vi "loadDataPerChannel.vi"(8 "error in (no error)":errorcluster, 10 "data":dbl[][][](array[numeric]), 11 "K2602 in":refnum<class "K2602.lvclass">) -> (0 "error out":errorcluster, 3 "K2602 out":refnum<class "K2602.lvclass">)   [LabVIEW 2009, in "Hardware.lvlib" / "Channels.lvlib" / "K2602.lvclass"]
uses:
  K2602.lvclass
  K2602.lvclass/K2602.ctl
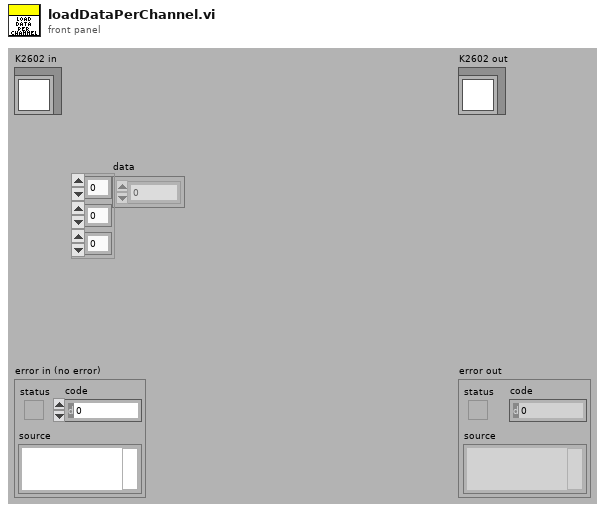
[diagram p1: front panel]
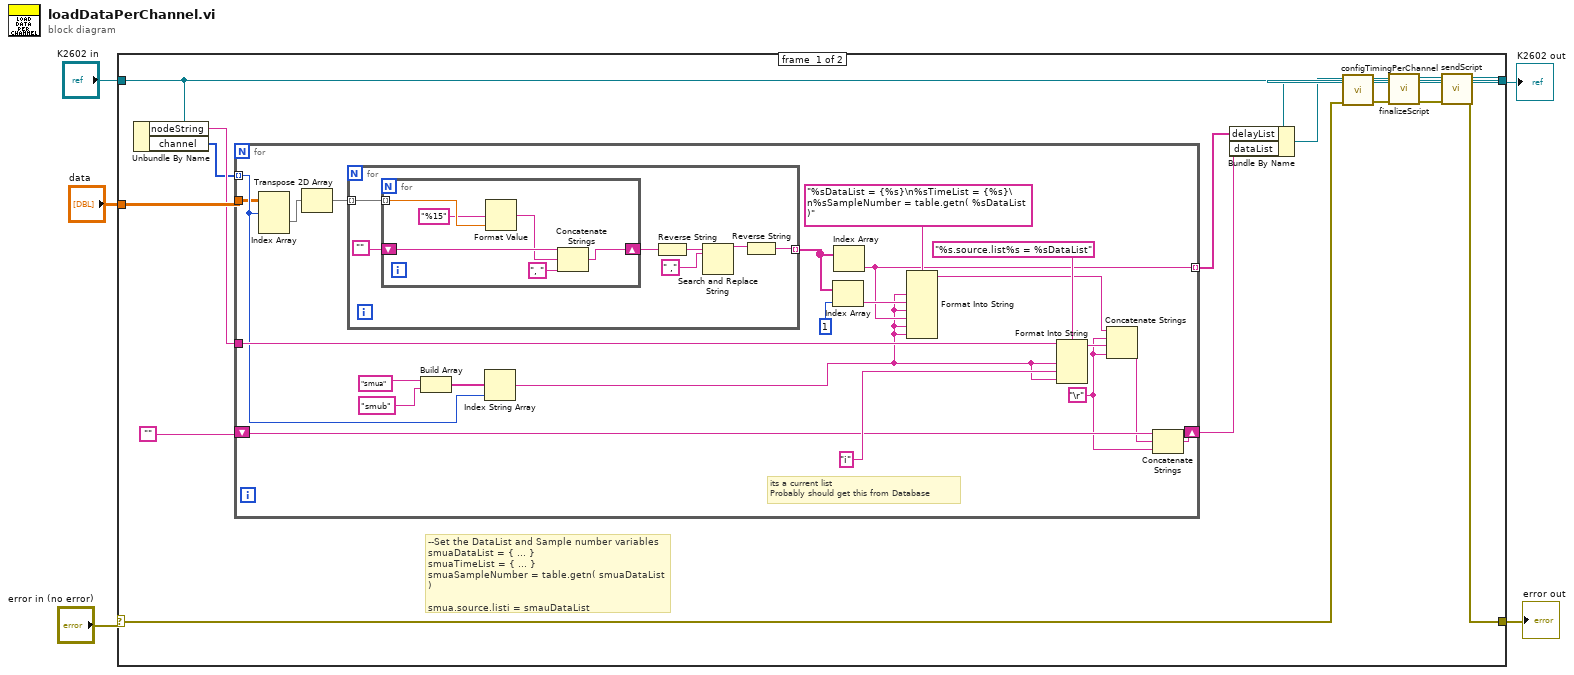
[diagram p0: block diagram]
diagram:
  n1 = case shown="No Error" "error in (no error)" {
    selector: "error in (no error)" -> [w13 w56]
    tunnel: [w7 w56] -> w4
    tunnel: [w8 w57] -> w2
    tunnel: "K2602 in" -> [w18 w57]
    tunnel: "data" -> [w20 _]
    frame #0 {
      # "--Set the DataList and Sample number variables\nsmuaDataList = { ... }\nsmuaTimeList = { ... }\nsmuaSampleNumber = table.getn( smuaDataList ) \n\nsmua.source.listi = smauDataList"
      n2 = Unbundle By Name(w18) -> ("nodeString"=w19:string, "channel"=w6:i32[])
      n3 = for {
        tunnel: w20 -> [w22]
        tunnel: w19 -> [w39]
        tunnel: [w27] -> w17 mode=indexing
        shift-right: [w34] -> w15
        shift-left: "" -> [w33]
        tunnel: w6 -> [w23] mode=indexing
        w24 = "\r"
        # "its a current list\nProbably should get this from Database"
        n4 = Index Array(array=w22, index (dim 0)=w23) -> (element=w21:dbl[][])  [unwired: 2 in]
        n5 = Transpose 2D Array(2D array=w21) -> (transposed array=w25:dbl[][])
        n6 = for {
          tunnel: w25 -> [w49] mode=indexing
          tunnel: [w43] -> w35 mode=indexing
          n7 = for {
            tunnel: w49 -> [w55] mode=indexing
            shift-right: [w50] -> w47
            shift-left: "" -> [w53]
            n8 = Format Value(format string="%15", value (0)=w55) -> (output string=w52:string)  [unwired: 1 in]
            n9 = Concatenate Strings(w53, w52, ", ") -> (w50:string)
          }
          n10 = Reverse String(1:w47) -> (0:w46:string)
          n11 = Search and Replace String(input string=w46, search string=" ,") -> (result string=w44:string)  [unwired: 6 in, 3 out]
          n12 = Reverse String(1:w44) -> (0:w43:string)
        }
        n13 = Build Array("smua", "smub") -> (w40:string[])
        n14 = Index String Array(1:w23, 2:w40) -> (0:w26:string)  [unwired: 1 in]
        n15 = Index Array(array=w35, index=1) -> (element=w31:string)
        n16 = Index Array(array=w35) -> (element=w27:string)  [unwired: 1 in]
        n17 = Format Into String(format string="%sDataList = {%s}\n%sTimeList = {%s}\n%sSampleNumber = table.getn( %sDataList )", w26, w31, w26, w27, w26, w26) -> (resulting string=w29:string)  [unwired: 2 in, 1 out]
        n18 = Format Into String(format string="%s.source.list%s = %sDataList", initial string=w39, w26, "i", w26) -> (resulting string=w28:string)  [unwired: 1 in, 1 out]
        n19 = Concatenate Strings(w29, w24, w28, w24) -> (w32:string)
        n20 = Concatenate Strings(w33, w32, w24) -> (w34:string)
      }
      n21 = Bundle By Name(cluster=w18, "delayList"=w17, "dataList"=w15) -> (w14:refnum<class "K2602.lvclass">)
      n22 = call-dynamic "configTimingPerChannel.vi"("error in (no error)"=w13, "K2602 in"=w14) -> ("error out"=w11:errorcluster, "K2602 out"=w12:refnum<class "K2602.lvclass">)  [unwired: 8 in]
      n23 = call "finalizeScript.vi"("error in (no error)"=w11, "K2602 in"=w12) -> ("error out"=w9:errorcluster, "K2602 out"=w10:refnum<class "K2602.lvclass">)  [unwired: 7 in, 1 out]
      n24 = call "sendScript.vi"("error in (no error)"=w9, "K2602 in"=w10) -> ("error out"=w7:errorcluster, "K2602 out"=w8:refnum<class "K2602.lvclass">)  [unwired: 8 in]
    }
    frame #1 {
    }
  }
  "error out" <- w4
  "K2602 out" <- w2
